vi "开关量输入状态解析.vi"(11 "输入字符串":string) -> (3 "开关量输入状态解析":T1)   [LabVIEW 2016, in "环境动力监测库.lvlib" / "空调库.lvlib"]
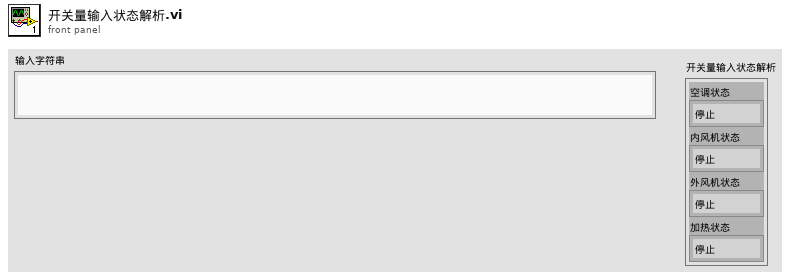
[diagram p1: front panel]
types:
  T1 = cluster{"空调状态":enum16{"停止", "运行"}, "内风机状态":enum16{"停止", "运行"}, "外风机状态":enum16{"停止", "运行"}, "加热状态":enum16{"停止", "运行"}}
  T2 = cluster{"空调状态":u16, "内风机状态":u16, "外风机状态":u16, "加热状态":u16}
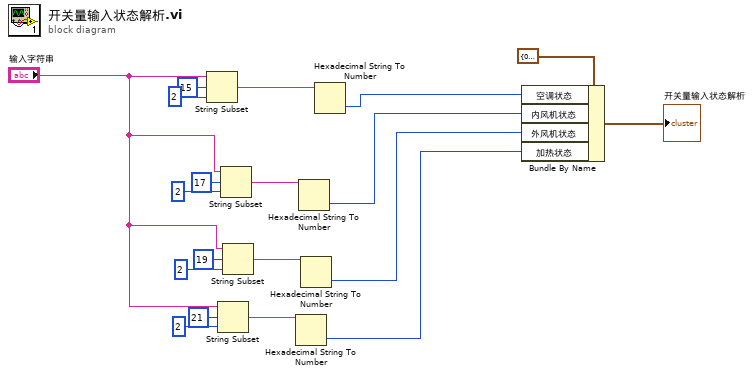
[diagram p0: block diagram]
diagram:
  n1 = String Subset(string="输入字符串", offset (0)=15 ("偏移量(0)"), length (rest)=2 ("长度（剩余）")) -> (substring=w17:string)
  n2 = String Subset(string="输入字符串", offset (0)=21 ("偏移量(0)"), length (rest)=2 ("长度（剩余）")) -> (substring=w8:string)
  n3 = String Subset(string="输入字符串", offset (0)=17 ("偏移量(0)"), length (rest)=2 ("长度（剩余）")) -> (substring=w14:string)
  n4 = String Subset(string="输入字符串", offset (0)=19 ("偏移量(0)"), length (rest)=2 ("长度（剩余）")) -> (substring=w13:string)
  n5 = Hexadecimal String To Number(string=w8) -> (number=w3:u32)  [unwired: 2 in, 1 out]
  n6 = Hexadecimal String To Number(string=w14) -> (number=w5:u32)  [unwired: 2 in, 1 out]
  n7 = Hexadecimal String To Number(string=w13) -> (number=w4:u32)  [unwired: 2 in, 1 out]
  n8 = Hexadecimal String To Number(string=w17) -> (number=w6:u32)  [unwired: 2 in, 1 out]
  n9 = Bundle By Name(cluster=T2 {"空调状态"=0, "内风机状态"=0, "外风机状态"=0, "加热状态"=0} ("系统模拟量量化数据"), "空调状态"=w6, "内风机状态"=w5, "外风机状态"=w4, "加热状态"=w3) -> (→"开关量输入状态解析":T2)
